vi "get message.vi"(11 "failure in":T1 {"code" format="%.0x"}) -> (2 "message":string, 3 "failure out":T1 {"code" format="%.0x"})   [LabVIEW 2013, in "failure.lvlib"]
uses:
  failure.lvlib
  failure.ctl
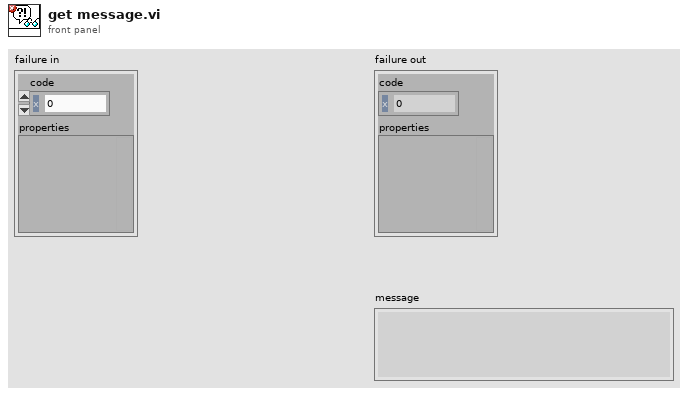
[diagram p1: front panel]
types:
  T1 = typedef "failure.lvlib/failure.ctl" = cluster{"code":i32, "properties":variant}
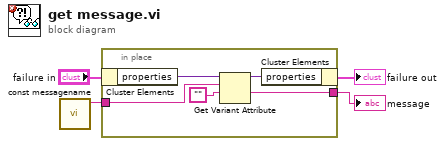
[diagram p0: block diagram]
diagram:
  n1 = call "const messagename.vi"() -> ("label"=w2:string)  [unwired: 11 in]
  n2 = in-place {
    in-place-border: w2 -> [w7]
    in-place-border: [w6] -> w1
    n3 = in-place-cluster #1("failure in") -> ("properties"=w9:variant)
    n4 = Get Variant Attribute(Variant=w9, name=w7, default value (empty Variant)="") -> (duplicate Variant=w8:variant, value=w6:string)  [unwired: 1 in, 2 out]
    n5 = in-place-cluster #1("properties"=w8) -> (→"failure out":T1)
  }
  "message" <- w1
